vi "ttm_aecontrol_poller.vi"(9 "silentRampRate":dbl, 10 "aeRampRate":dbl) -> ()   [LabVIEW 2009]
panel:
  out "Number of points":i32=1000
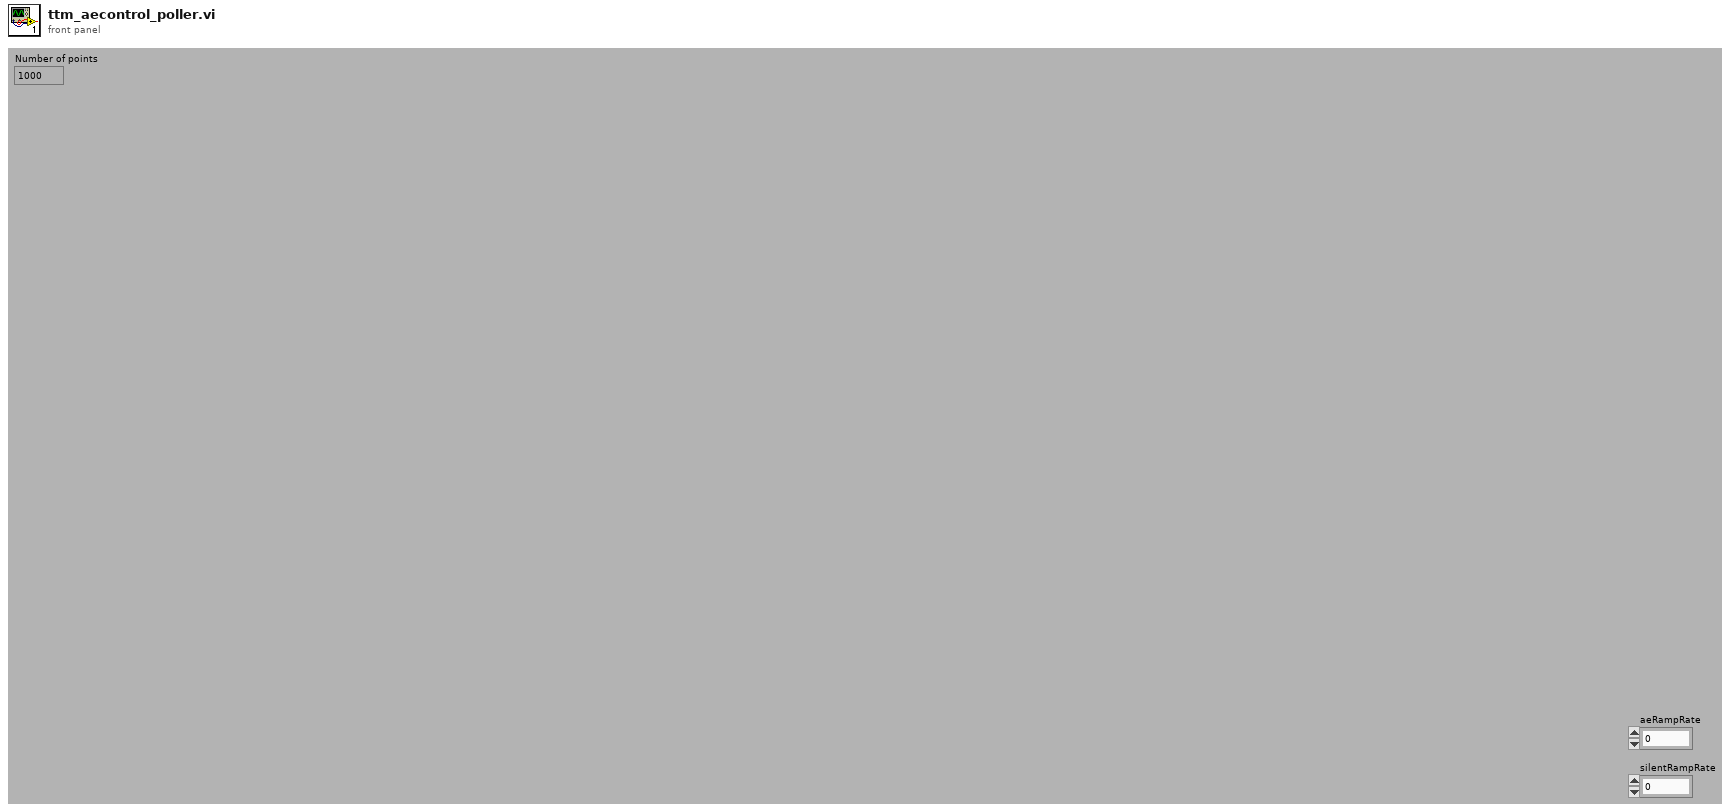
[diagram p1: front panel]
types:
  T1 = cluster{"Data Sample Format (0)":i8, "Loop code (2)":i8, "Target Amplitude (32767)":i16, "Playback rate":dbl, "Playback Scale":dbl[], "Envelope Ramp Rate":dbl, "Filter Order (0)":i8, "Filter Type (0)":i8, "Filter Bandwidth":dbl}
  T2 = cluster{"Name":string, "Type":i32, "SI Full Scale":dbl, "Full Scale":dbl, "Units String":string, "Display Format":string, "Gauge Length":dbl}[][]
  T3 = cluster{"Device ID":i32, "Device Name":string, "Device Type":i32}[]
  T4 = cluster{"Axis Information Out[0]":cluster{"Device ID":i32, "Device Name":string, "Device Type":i32}, "Axis Information Out[1]":cluster{"Device ID":i32, "Device Name":string, "Device Type":i32}, "Axis Information Out[2]":cluster{"Device ID":i32, "Device Name":string, "Device Type":i32}, "Axis Information Out[3]":cluster{"Device ID":i32, "Device Name":string, "Device Type":i32}, "Axis Information Out[4]":cluster{"Device ID":i32, "Device Name":string, "Device Type":i32}, "Axis Information Out[5]":cluster{"Device ID":i32, "Device Name":string, "Device Type":i32}, "Axis Information Out[6]":cluster{"Device ID":i32, "Device Name":string, "Device Type":i32}, "Axis Information Out[7]":cluster{"Device ID":i32, "Device Name":string, "Device Type":i32}, "Axis Information Out[8]":cluster{"Device ID":i32, "Device Name":string, "Device Type":i32}}
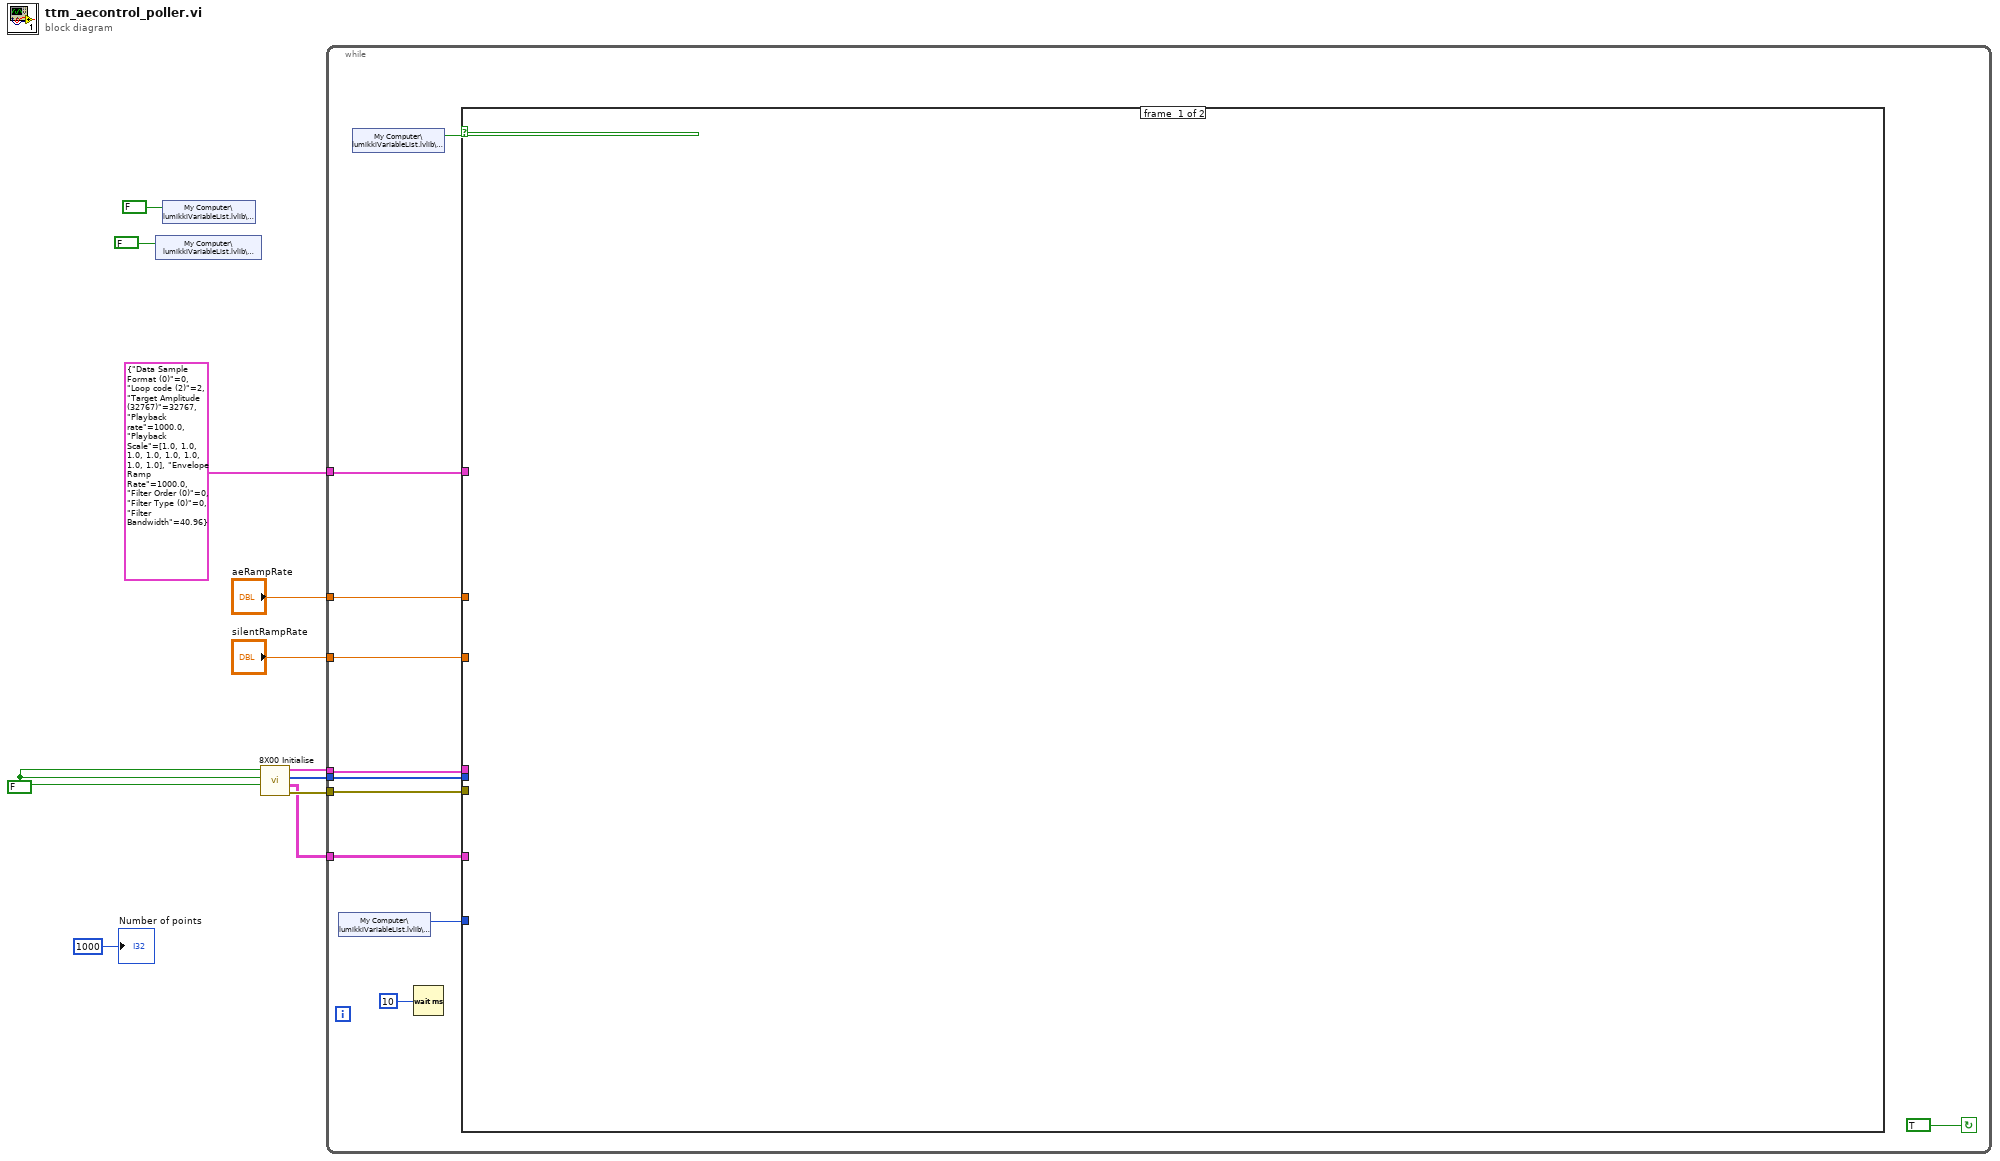
[diagram p0: block diagram]
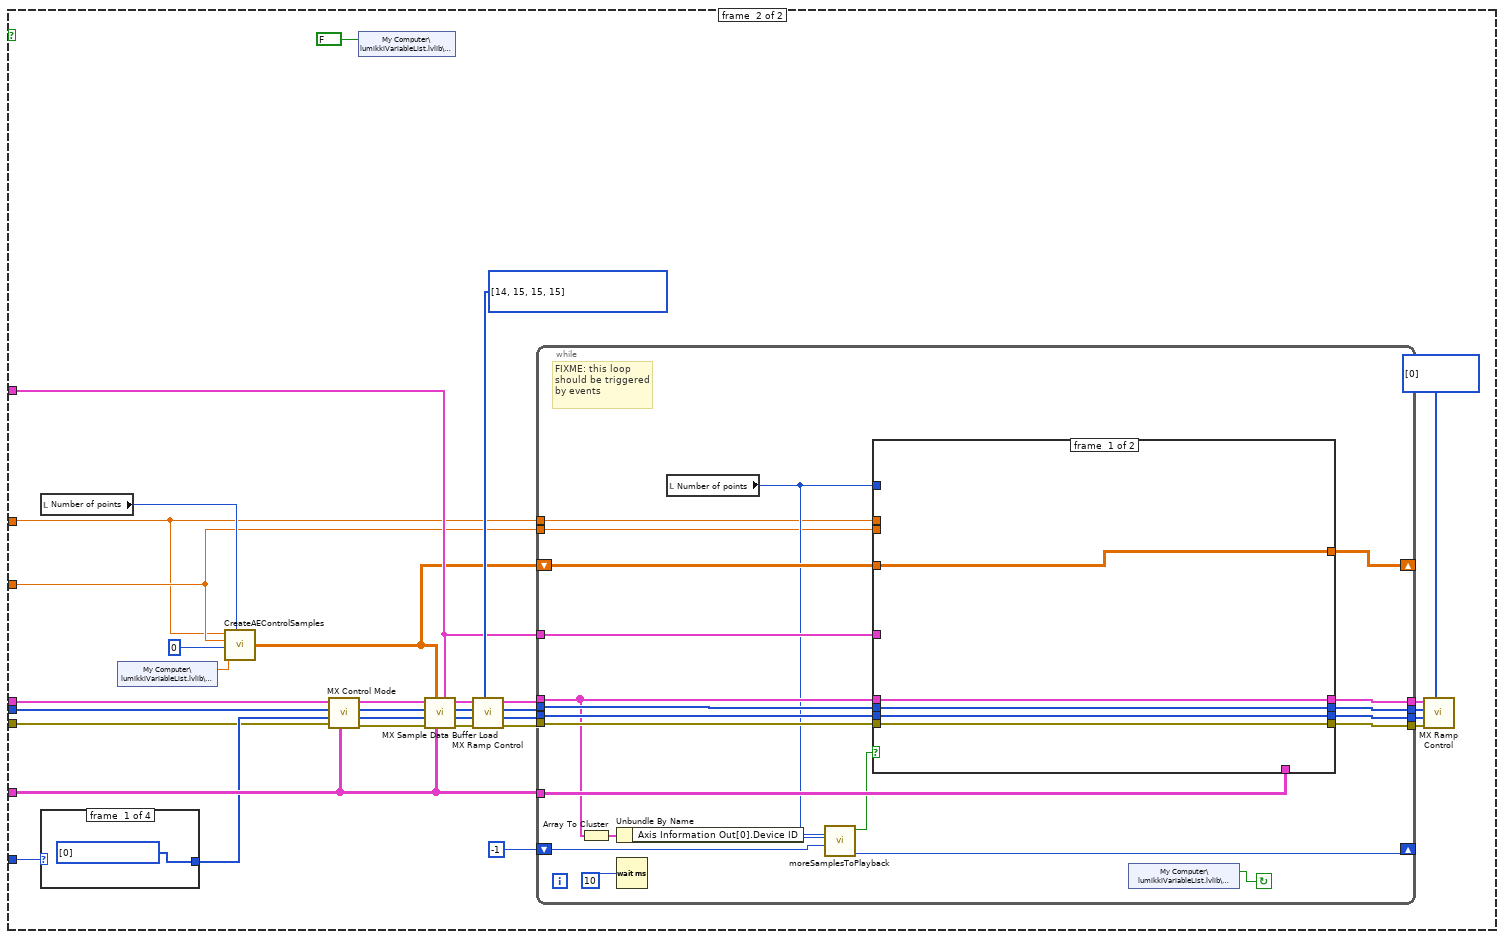
[diagram p2: hidden frame]
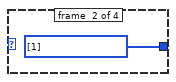
[diagram p3: hidden frame]
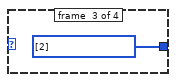
[diagram p4: hidden frame]
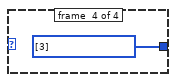
[diagram p5: hidden frame]
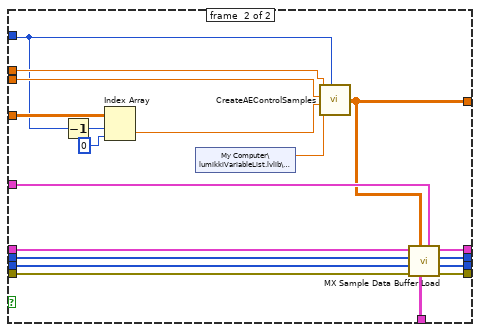
[diagram p6: hidden frame]
diagram:
  w8 = FALSE ("Reset")
  n1 = shared-variable "My Computer\\lumikkiVariableList.lvlib\\creepRunning"(FALSE ("startCreep")) -> ()  [unwired: 1 in, 1 out]
  n2 = shared-variable "My Computer\\lumikkiVariableList.lvlib\\startCreep"(FALSE ("startCreep")) -> ()  [unwired: 1 in, 1 out]
  n3 = call "8X00 Initialise.vi"("Reset?"=w8, "Create DVM? (T)"=w8, "Create Console? (T)"=w8) -> ("error out"=w11:errorcluster, "Channel Data"=w10:T2, "Axis Selector"=w7:i32[], "Axis Information"=w9:T3)  [unwired: 1 in]
  n4 = while {
    tunnel: w10 -> [w22]
    tunnel: w9 -> [w18]
    tunnel: w11 -> [w16]
    tunnel: w7 -> [w17]
    tunnel: T1 {"Data Sample Format (0)"=0, "Loop code (2)"=2, "Target Amplitude (32767)"=32767, "Playback rate"=1000.0, "Playback Scale"=[1.0, 1.0, 1.0, 1.0, 1.0, 1.0, 1.0, 1.0], "Envelope Ramp Rate"=1000.0, "Filter Order (0)"=0, "Filter Type (0)"=0, "Filter Bandwidth"=40.96} ("Sample Data Playback Definition") -> [w14]
    tunnel: "aeRampRate" -> [w13]
    tunnel: "silentRampRate" -> [w12]
    stop <- TRUE continue-if-true
    n5 = shared-variable "My Computer\\lumikkiVariableList.lvlib\\channelInt"() -> (w15:i32)  [unwired: 1 in, 1 out]
    n6 = shared-variable "My Computer\\lumikkiVariableList.lvlib\\startCreep"() -> (w19:bool)  [unwired: 1 in, 1 out]
    n7 = Wait (ms)(milliseconds to wait=u32 10) -> ()  [unwired: 1 out]
    n8 = case shown="True" w19 {
      tunnel: w22 -> [_ w39]
      tunnel: w18 -> [_ w34]
      tunnel: w17 -> [_ w33]
      tunnel: w16 -> [_ w31]
      tunnel: w15 -> [_ w45]
      tunnel: w14 -> [_ w30]
      tunnel: w13 -> [_ w23]
      tunnel: w12 -> [_ w24]
      frame #0 {
      }
      frame #1 {
        w40 = u16[] [0] items=["Stop", "Start or continue", "Hold", "Continue", "Return ramp to set level at fixed rate", "Reserved", "Reserved", "Start Random without demand hold", "Start Random with demand hold", "Prepare Random Start without demand hold", "Prepare Random Start with demand hold", "Unslave", "Reserved", "Reserved", "Start Sample Data Playback or Resume", "Prepare for Start of Sample Data", "Reserved", "Reserved", "Resume Playback", "Start an electromechanical frame return"] ("Ramp Control")
        w51 = u16[] [14, 15, 15, 15] items=["Stop", "Start or continue", "Hold", "Continue", "Return ramp to set level at fixed rate", "Reserved", "Reserved", "Start Random without demand hold", "Start Random with demand hold", "Prepare Random Start without demand hold", "Prepare Random Start with demand hold", "Unslave", "Reserved", "Reserved", "Start Sample Data Playback or Resume", "Prepare for Start of Sample Data", "Reserved", "Reserved", "Resume Playback"] ("Ramp Control")
        n9 = local read "Number of points"() -> (w27:i32)
        n10 = case shown="2" w45 {
          tunnel: [w56 w57 w58 w59] -> w32
          frame #0 {
            w56 = u16[] [0] items=["Channel 1", "Channel 2", "Channel 3", "Channel 4"] ("Choose channel to apply\nthe setpoint")
          }
          frame #1 {
            w57 = u16[] [1] items=["Channel 1", "Channel 2", "Channel 3", "Channel 4"] ("Choose channel to apply\nthe setpoint")
          }
          frame #2 {
            w58 = u16[] [2] items=["Channel 1", "Channel 2", "Channel 3", "Channel 4"] ("Choose channel to apply\nthe setpoint")
          }
          frame #3 {
            w59 = u16[] [3] items=["Channel 1", "Channel 2", "Channel 3", "Channel 4"] ("Choose channel to apply\nthe setpoint")
          }
        }
        n11 = shared-variable "My Computer\\lumikkiVariableList.lvlib\\AEdataSum"() -> (w25:dbl)  [unwired: 1 in, 1 out]
        n12 = call "CreateAEControlSamples.vi"("aeRampRate"=w23, "silentRampRate"=w24, "initialOrPreviousStrain"=0, "AEdataSum"=w25, "outputLength"=w27) -> ("output array"=w28:dbl[][])
        n13 = call "MX Control Mode.vi"("Channel Data"=w39, "error in (no error)"=w31, "Control Modes"=w32, "Axis Selector"=w33, "Axis Information"=w34) -> ("error out"=w35:errorcluster, "Control Modes out"=w36:u16[], "Axis Selector out"=w37:i32[], "Axis Information out"=w38:T3)  [unwired: 1 in]
        n14 = shared-variable "My Computer\\lumikkiVariableList.lvlib\\startCreep"(FALSE ("startCreep")) -> ()  [unwired: 1 in, 1 out]
        n15 = call "MX Sample Data Buffer Load.vi"("Sample Data Playback Definition"=w30, "Channel Data"=w39, "Sample Data"=w28, "error in (no error)"=w35, "Channels In"=w36, "Axis Selector In"=w37, "Axis Information In"=w38) -> ("error out"=w53:errorcluster, "Channels Out"=w52:u16[], "Axis Selector Out"=w54:i32[], "Axis Information Out"=w55:T3)  [unwired: 1 in]
        n16 = call "MX Ramp Control.vi"("Ramp Control"=w51, "error in (no error)"=w53, "Channels In"=w52, "Axis Selector In"=w54, "Axis Information In"=w55) -> ("error out"=w48:errorcluster, "Channels Out"=w50:u16[], "Axis Selector Out"=w49:i32[], "Axis Information Out"=w47:T3)  [unwired: 2 in]
        n17 = while {
          tunnel: w47 -> [w70]
          tunnel: w49 -> [w81]
          tunnel: w50 -> [w74]
          tunnel: w48 -> [w80]
          tunnel: [w71] -> w44
          tunnel: [w79] -> w43
          tunnel: [w78] -> w42
          tunnel: [w77] -> w41
          tunnel: w30 -> [w69]
          tunnel: w39 -> [w76]
          shift-right: [w63] -> _
          shift-left: w28 -> [w65]
          shift-right: [w67] -> _
          shift-left: -1 -> [w66]
          tunnel: w24 -> [w61]
          tunnel: w23 -> [w60]
          stop <- w75 continue-if-true
          # "FIXME: this loop \nshould be triggered \nby events"
          n18 = Array To Cluster(array=w70) -> (cluster=w72:T4)
          n19 = Unbundle By Name(w72) -> ("Axis Information Out[0].Device ID"=w68:i32)
          n20 = Wait (ms)(milliseconds to wait=u32 10) -> ()  [unwired: 1 out]
          n21 = local read "Number of points"() -> (w64:i32)
          n22 = call "moreSamplesToPlayback.vi"("Device"=w68, "playbackCycleLength"=w64, "previousSampleCycle"=w66) -> ("ReadyForMore"=w62:bool, "currentSampleCycle"=w67:i32)  [unwired: 6 in]
          n23 = case shown="True" w62 {
            tunnel: w81 -> [w85 w105]
            tunnel: w80 -> [w83 w104]
            tunnel: [w85 w103] -> w79
            tunnel: [w84 w102] -> w78
            tunnel: [w83 w101] -> w77
            tunnel: w69 -> [_ w100]
            tunnel: w76 -> [_ w99]
            tunnel: w74 -> [w84 w98]
            tunnel: [w86 w97] -> w71
            tunnel: w70 -> [w86 w96]
            tunnel: w65 -> [w82 w93]
            tunnel: w64 -> [_ w87]
            tunnel: [w82 w92] -> w63
            tunnel: w61 -> [_ w89]
            tunnel: w60 -> [_ w88]
            frame #0 {
            }
            frame #1 {
              n24 = Decrement(x=w87) -> (x-1=w95:i32)
              n25 = Index Array(array=w93, index (row)=w95, index (col)=0) -> (element=w91:dbl)
              n26 = shared-variable "My Computer\\lumikkiVariableList.lvlib\\AEdataSum"() -> (w90:dbl)  [unwired: 1 in, 1 out]
              n27 = call "CreateAEControlSamples.vi"("aeRampRate"=w88, "silentRampRate"=w89, "initialOrPreviousStrain"=w91, "AEdataSum"=w90, "outputLength"=w87) -> ("output array"=w92:dbl[][])
              n28 = call "MX Sample Data Buffer Load.vi"("Sample Data Playback Definition"=w100, "Channel Data"=w99, "Sample Data"=w92, "error in (no error)"=w104, "Channels In"=w98, "Axis Selector In"=w105, "Axis Information In"=w96) -> ("error out"=w101:errorcluster, "Channels Out"=w102:u16[], "Axis Selector Out"=w103:i32[], "Axis Information Out"=w97:T3)  [unwired: 1 in]
            }
          }
          n29 = shared-variable "My Computer\\lumikkiVariableList.lvlib\\creepRunning"() -> (w75:bool)  [unwired: 1 in, 1 out]
        }
        n30 = call "MX Ramp Control.vi"("Ramp Control"=w40, "error in (no error)"=w41, "Channels In"=w42, "Axis Selector In"=w43, "Axis Information In"=w44) -> ()  [unwired: 2 in, 4 out]
      }
    }
  }
  "Number of points" <- 1000 ("Number of points")
